vi "Set Sys Cfgs.vi"(8 "error in (no error)":errorcluster, 9 "sys cfgs":refnum<class "[V] Sys Cfg Base.lvclass">[](array[class]), 10 "names":string[](array[string]), 11 "[V] Sys Cfg Main in":refnum<class "[V] Sys Cfg Main.lvclass">) -> (0 "error out":errorcluster, 3 "[V] Sys Cfg Main out":refnum<class "[V] Sys Cfg Main.lvclass">)   [LabVIEW 2020, in "[V] Sys Cfg Main.lvlib" / "[V] Sys Cfg Main.lvclass"]
uses:
  [V] Sys Cfg Main.lvclass
  [V] Sys Cfg Base/[V] Sys Cfg Base/[V] Sys Cfg Base.lvclass
  [V] Sys Cfg Main.lvclass/[V] Sys Cfg Main.ctl
  [V] Sys Cfg Base/[V] Sys Cfg Base/[V] Sys Cfg Base.lvclass/[V] Sys Cfg Base.ctl
  [V] Sys Cfg Base/[V] Sys Cfg Base/Accessor/Write cfg file folder.vi
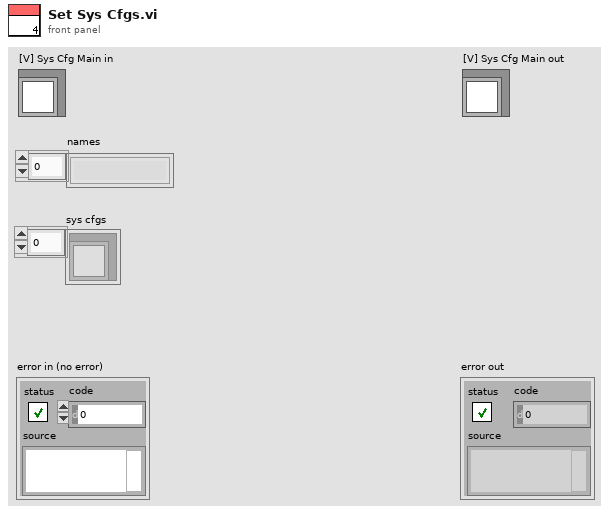
[diagram p1: front panel]
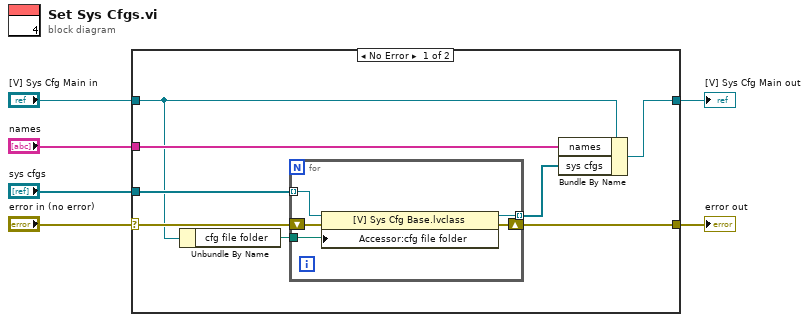
[diagram p0: block diagram]
diagram:
  n1 = case shown="No Error" "error in (no error)" {
    selector: "error in (no error)" -> [w13 w21]
    tunnel: [w7 w21] -> w5
    tunnel: [w8 w20] -> w3
    tunnel: "[V] Sys Cfg Main in" -> [w11 w20]
    tunnel: "names" -> [w14 _]
    tunnel: "sys cfgs" -> [w12 _]
    frame No Error {
      n2 = Unbundle By Name(w11) -> ("cfg file folder"=w10:path)
      n3 = for {
        tunnel: w12 -> [w18] mode=indexing
        shift-right: [w17] -> w7
        shift-left: w13 -> [w19]
        tunnel: w10 -> [w16]
        tunnel: [w15] -> w9 mode=indexing
        n4 = property class="[V] Sys Cfg Base.lvclass"(reference=w18, error in=w19, "Accessor:cfg file folder"=w16) -> (reference out=w15:refnum<class "[V] Sys Cfg Base.lvclass">, error out=w17:errorcluster)
      }
      n5 = Bundle By Name(cluster=w11, "names"=w14, "sys cfgs"=w9) -> (w8:refnum<class "[V] Sys Cfg Main.lvclass">)
    }
    frame Error {
    }
  }
  "error out" <- w5
  "[V] Sys Cfg Main out" <- w3
